vi "sub vi - AI USB4704 (3) v7.vi"() -> (1 "Graph 1":dynamicdata(graph), 2 "Graph 2":dynamicdata(graph), 3 "Graph 3":dynamicdata(graph), 10 "loop time":dbl format="%.6g", 15 "error array":errorcluster[](array[cluster]))   [LabVIEW 2013]
uses:
  program files/Global 1.vi
panel:
  in  "Tab Control":enum32{"Page 1", "Page 2", "Page 3"}(tab)
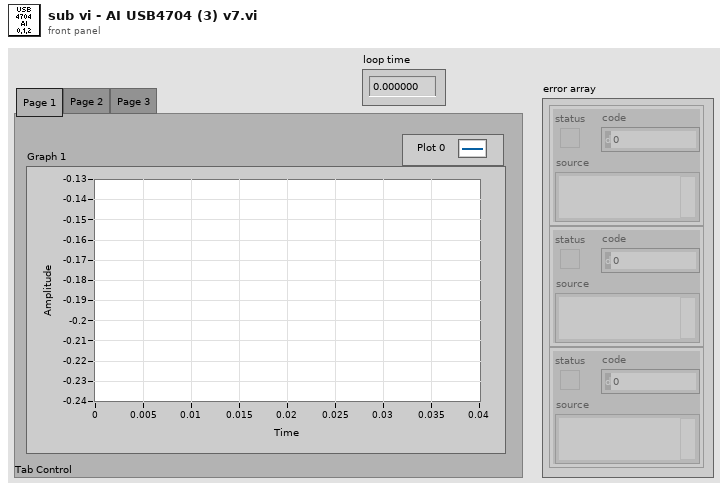
[diagram p1: front panel]
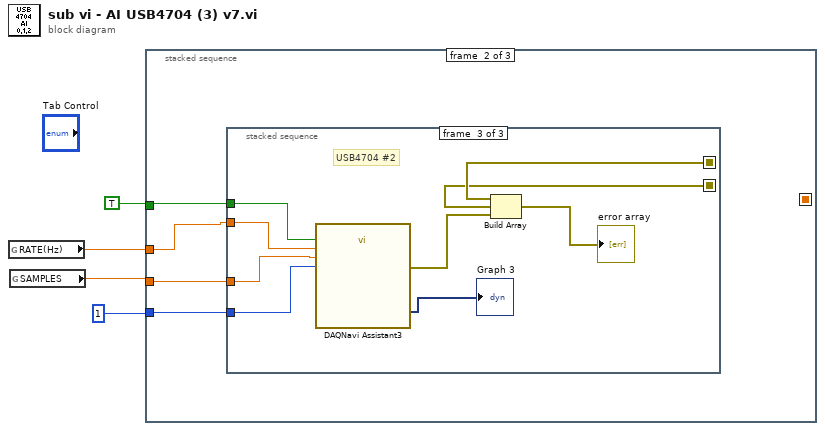
[diagram p0: block diagram]
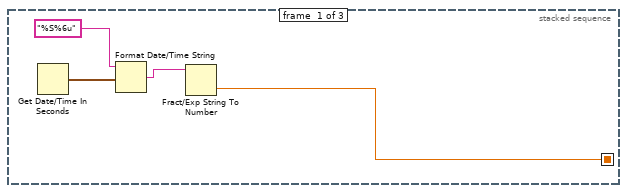
[diagram p2: hidden frame]
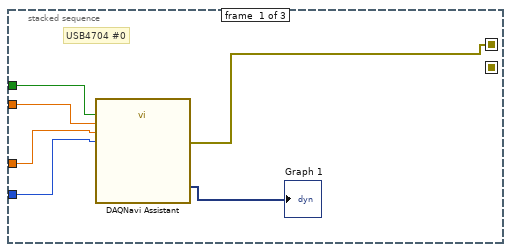
[diagram p3: hidden frame]
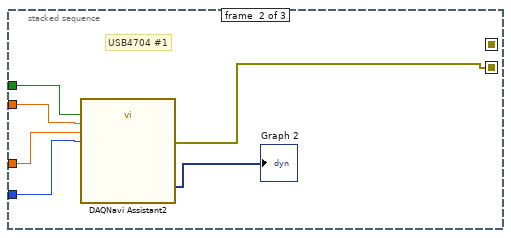
[diagram p4: hidden frame]
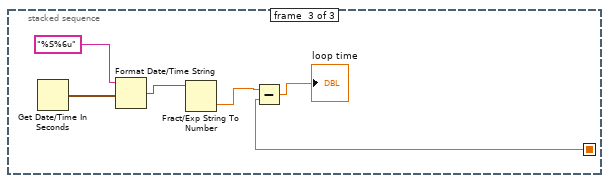
[diagram p5: hidden frame]
diagram:
  n1 = global read "Global 1.vi" "RATE(Hz)"() -> (w2:dbl)
  n2 = global read "Global 1.vi" "SAMPLES"() -> (w1:dbl)
  n3 = stacked-sequence {
    seq-local: [w5 _ _] -> [_ _ w35]
    tunnel: TRUE -> [_ w12 _]
    tunnel: 1 -> [_ w10 _]
    tunnel: w1 -> [_ w11 _]
    tunnel: w2 -> [_ w9 _]
    frame #0 {
      n4 = Get Date/Time In Seconds() -> (seconds since 1Jan1904=w7:timestamp)
      n5 = Format Date/Time String(time format string (%c)="%S%6u", seconds (now)=w7) -> (date/time string=w6:string)  [unwired: 1 in]
      n6 = Fract/Exp String To Number(string=w6) -> (number=w5:dbl)  [unwired: 3 in, 1 out]
    }
    frame #1 {
      n7 = stacked-sequence {
        seq-local: [w14 _ _] -> [_ _ w33]
        seq-local: [_ w20 _] -> [_ _ w32]
        tunnel: w12 -> [w18 w24 w30]
        tunnel: w9 -> [w17 w23 w29]
        tunnel: w11 -> [w16 w22 w28]
        tunnel: w10 -> [w15 w21 w27]
        frame #0 {
          # "USB4704 #0"
          n8 = call "DAQNavi Assistant"("stop(true)"=w18, "conversion rate(Hz)"=w17, "samples"=w16, "time out(10s)"=w15) -> ("error out"=w14:errorcluster, "data out(DDT)"=→"Graph 1":dynamicdata)  [unwired: 22 in]
        }
        frame #1 {
          # "USB4704 #1"
          n9 = call "DAQNavi Assistant2"("stop(true)"=w24, "conversion rate(Hz)"=w23, "samples"=w22, "time out(10s)"=w21) -> ("error out"=w20:errorcluster, "data out(DDT)"=→"Graph 2":dynamicdata)  [unwired: 22 in]
        }
        frame #2 {
          # "USB4704 #2"
          n10 = call "DAQNavi Assistant3"("stop(true)"=w30, "conversion rate(Hz)"=w29, "samples"=w28, "time out(10s)"=w27) -> ("error out"=w26:errorcluster, "data out(DDT)"=→"Graph 3":dynamicdata)  [unwired: 22 in]
          n11 = Build Array(w33, w32, w26) -> (→"error array":errorcluster[])
        }
      }
    }
    frame #2 {
      n12 = Get Date/Time In Seconds() -> (seconds since 1Jan1904=w38:timestamp)
      n13 = Format Date/Time String(time format string (%c)="%S%6u", seconds (now)=w38) -> (date/time string=w37:string)  [unwired: 1 in]
      n14 = Fract/Exp String To Number(string=w37) -> (number=w36:dbl)  [unwired: 3 in, 1 out]
      n15 = Subtract(x=w36, y=w35) -> (x-y=→"loop time":dbl)
    }
  }
